vi "Close.vi"(8 "error in (no error)":errorcluster, 10 "Msg in":T1, 11 "FakePressureController in":refnum<class "PXIDigitizer.lvclass">) -> (0 "error out":errorcluster, 1 "new command":string, 2 "Msg out":T1, 3 "FakePressureController out":refnum<class "PXIDigitizer.lvclass">)   [LabVIEW 2011, in "PXIDigitizer.lvclass"]
uses:
  PXIDigitizer.lvclass
  DriverMsg.ctl
  BaseDriver/BaseDriver.lvclass
  PXIDigitizer.lvclass/PXIDigitizer.ctl
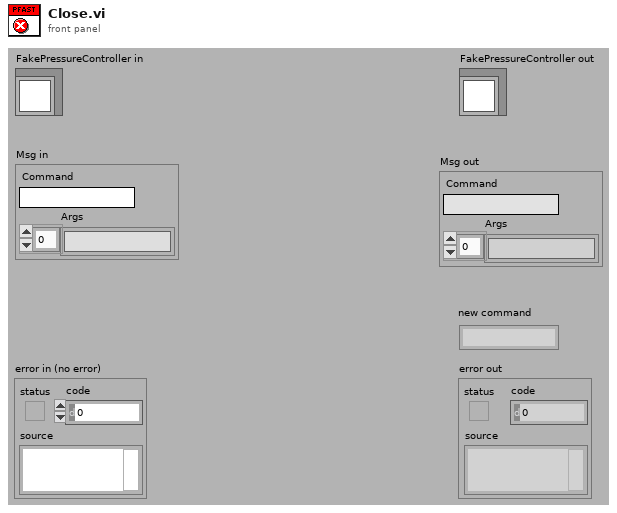
[diagram p1: front panel]
types:
  T1 = typedef "DriverMsg.ctl" = cluster{"Command":string, "Args":string[]}
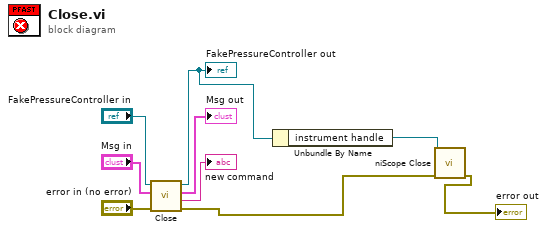
[diagram p0: block diagram]
diagram:
  n1 = call-parent "Close.vi"("error in (no error)"="error in (no error)", "Msg in"="Msg in", "BaseDriver in"="FakePressureController in") -> ("error out"=w2:errorcluster, "new command"=→"new command":string, "Msg out"=→"Msg out":T1, "BaseDriver out"=w4:refnum<class "PXIDigitizer.lvclass">)  [unwired: 5 in]
  "FakePressureController out" <- w4
  n2 = Unbundle By Name(w4) -> ("instrument handle"=w3:refnum<k15>)
  n3 = call "niScope Close.vi"("instrument handle"=w3, "error in"=w2) -> ("error out"=→"error out":errorcluster)  [unwired: 13 in]
